vi "Quary Mode.vi"(9 "error in (no error)":errorcluster, 10 "VISA resource name":refnum<visa-resource-name>) -> (0 "Mode":string, 1 "error out":errorcluster, 2 "VISA resource name out":refnum<visa-resource-name>)   [LabVIEW 2018]
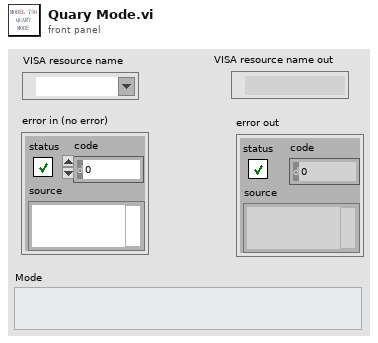
[diagram p1: front panel]
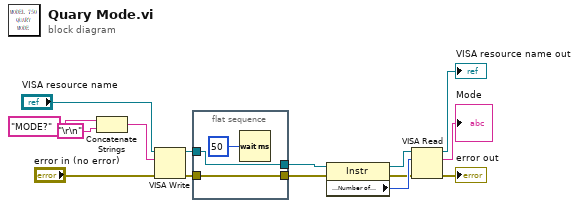
[diagram p0: block diagram]
diagram:
  n1 = Concatenate Strings("MODE?" ("字符串"), "\r\n") -> (w11:string)
  n2 = VISA Write(VISA resource name="VISA resource name", write buffer=w11, error in (no error)="error in (no error)") -> (VISA resource name out=w10:refnum<visa-resource-name>, error out=w9:errorcluster)  [unwired: 1 out]
  n3 = flat-sequence {
    tunnel: [w18] -> w6
    tunnel: w10 -> [w18]
    tunnel: [w17] -> w5
    tunnel: w9 -> [w17]
    frame #0 {
      n4 = Wait (ms)(milliseconds to wait=u32 50 ("等待时间（毫秒）")) -> ()  [unwired: 1 out]
    }
  }
  n5 = property class="Instr"(reference=w6, error in=w5) -> (reference out=w4:refnum<visa-resource-name>, error out=w2:errorcluster, "Serial Settings:Number of Bytes at Serial Port"=w3:u32)
  n6 = VISA Read(VISA resource name=w4, byte count=w3, error in (no error)=w2) -> (VISA resource name out=→"VISA resource name out":refnum<visa-resource-name>, read buffer=→"Mode":string, error out=→"error out":errorcluster)  [unwired: 1 out]
